vi "Check Flow Control.vi"(11 "payload":u8[](array[numeric]) format="%.0x") -> (2 "Block Size":u16 format="%.0x", 3 "Flow Control?":bool)   [LabVIEW 2018]
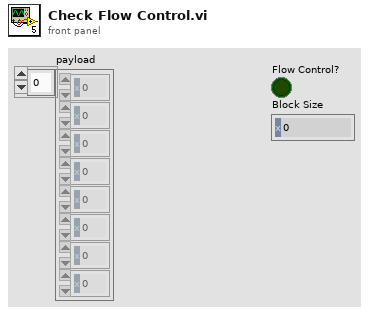
[diagram p1: front panel]
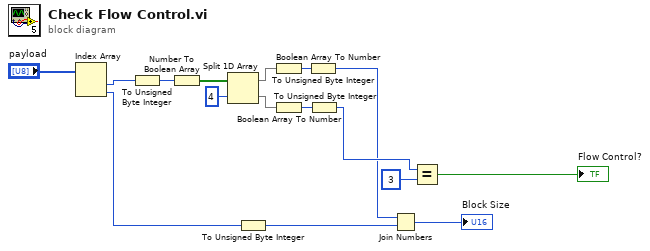
[diagram p0: block diagram]
diagram:
  n1 = Index Array(array="payload") -> (element #1=w7:u8, element #2=w6:u8)  [unwired: 2 in]
  n2 = To Unsigned Byte Integer(number=w7) -> (unsigned 8bit integer=w16:u8)
  n3 = Number To Boolean Array(number=w16) -> (Boolean array=w15:bool[])
  n4 = Split 1D Array(array=w15, index=4) -> (first subarray=w13:bool[], second subarray=w12:bool[])
  n5 = To Unsigned Byte Integer(number=w6) -> (unsigned 8bit integer=w4:u8)
  n6 = Boolean Array To Number(Boolean array=w13) -> (number=w5:u32)
  n7 = Boolean Array To Number(Boolean array=w12) -> (number=w11:u32)
  n8 = To Unsigned Byte Integer(number=w5) -> (unsigned 8bit integer=w1:u8)
  n9 = To Unsigned Byte Integer(number=w11) -> (unsigned 8bit integer=w2:u8)
  n10 = Join Numbers(hi=w1, lo=w4) -> ((hi.lo)=→"Block Size":u16)
  n11 = Equal?(x=w2, y=u32 3) -> (x = y?=→"Flow Control?":bool)
